vi "CCM-TDT-Read Connection Tables.vi"(0 "Path In":path, 7 "TDT-Device Config":T2, 11 "error in (no error)":errorcluster) -> (8 "Tables":cluster{"Table":T1[]}[](array[cluster]), 15 "error out":errorcluster)   [LabVIEW 2020]
uses:
  PXI DAQ VIs/TDT VIs/Typedefs/TDT-Device Config.ctl
  PXI DAQ VIs/TDT VIs/Typedefs/TDT-Output source.ctl
  PXI DAQ VIs/TDT VIs/Typedefs/TDT-Device ID.ctl
  PXI DAQ VIs/TDT VIs/Typedefs/TDT-Input source.ctl
  Type Defs/CM-Connection.ctl
panel:
  out "Path Out":path
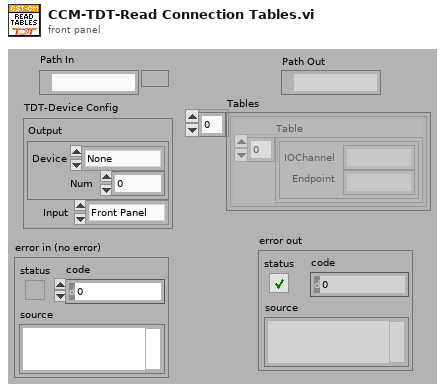
[diagram p1: front panel]
types:
  T1 = typedef "CM-Connection.ctl" = cluster{"IOChannel":string, "Endpoint":string}
  T2 = typedef "TDT-Device Config.ctl" = cluster{"Output":T3, "Input":T5}
  T3 = typedef "TDT-Output source.ctl" = cluster{"Device":T4, "Num":i32}
  T4 = typedef "TDT-Device ID.ctl" = enum16{"None", "PA5", "RP2", "RL2", "RA16", "RV8", "RX5", "RX6", "RX7", "RX8", "RZ2", "RZ5", "RZ6"}
  T5 = typedef "TDT-Input source.ctl" = enum16{"Front Panel", "RA4LI", "RA16LI"}
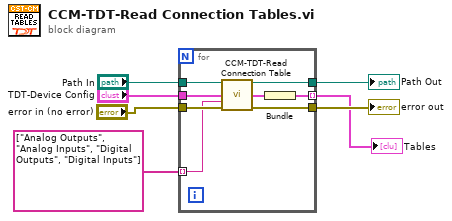
[diagram p0: block diagram]
diagram:
  n1 = for {
    tunnel: string[] ["Analog Outputs", "Analog Inputs", "Digital Outputs", "Digital Inputs"] -> [w12] mode=indexing
    tunnel: "Path In" -> [w15]
    tunnel: "TDT-Device Config" -> [w14]
    tunnel: "error in (no error)" -> [w13]
    tunnel: [w11] -> w3
    tunnel: [w10] -> w2
    tunnel: [w9] -> w1 mode=indexing
    n2 = call "CCM-TDT-Read Connection Table.vi"("Path In"=w15, "TDT-Device Config"=w14, "Type"=w12, "error in (no error)"=w13) -> ("Path Out"=w11:path, "Table"=w8:T1[], "error out"=w10:errorcluster)  [unwired: 9 in]
    n3 = Bundle("Table"=w8) -> (w9:cluster{"Table":T1[]})  [unwired: 1 in]
  }
  "error out" <- w2
  "Path Out" <- w3
  "Tables" <- w1
